vi "Begin.vi"(8 "error in":errorcluster) -> (0 "error out":errorcluster)   [LabVIEW 2018]
doc: "Called before other user functions, this VI is expected to open initial I/O refnums, load in file data, and do all program initialization. Notice that the <B>error out</B> terminal is simply used for data flow. Wiring it to other structures or subVIs ensures that this VI runs first."
uses:
  <vilib>/Rock Robotics/WPI/DriverStation/WPI_DriverStationRobotMode2.ctl
  <vilib>/Rock Robotics/WPI/Joystick/WPI_JoystickDeviceEnum.ctl
  Robot Global Data.vi
  <vilib>/Rock Robotics/Network Tables/NT Write String Array.vi
  <vilib>/Rock Robotics/WPI/RobotDrive/WPI_RobotDriveOpen2MotorWithExistingMotors.vi
  <vilib>/Rock Robotics/SystemInterfaces/DIO/FPGA_DIOPWMChannel.ctl
  <vilib>/Rock Robotics/WPI/SafetyOutput/WPI_SafetyOutputConfigMenu.ctl
  <vilib>/Rock Robotics/WPI/RobotDrive/WPI_RobotDriveOpen4MotorWithTalon.vi
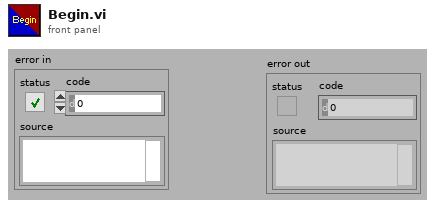
[diagram p1: front panel]
types:
  T1 = enum16{"Talon-RightDrive", "Victor-Right1", "Victor-Right2", "Talon-RHabArm", "Talon-RHabSlide", "Victor-CargoIntake1", "Victor-CargoIntake2", "Talon-CargoRotate", "Empty1", "Empty2", "Victor-HabWheel", "Talon-LHabSlide", "Talon-LHabArm", "Victor-Left1", "Victor-Left2", "Talon-LeftDrive"}
  T2 = typedef "WPI_JoystickDeviceEnum.ctl" = enum16{"USB 0", "USB 1", "USB 2", "USB 3", "USB 4", "USB 5"}
  T3 = typedef "WPI_DriverStationRobotMode2.ctl" = enum16{"Autonomous Disabled", "Autonomous Enabled", "Teleop Disabled", "Teleop Enabled", "Disconnected", "Finish", "Test Disabled", "Test Enabled", "Emergency Stopped"}
  T4 = typedef "CTRE_CANifier_PWMChannel.ctl" = enum16{"PWMChannel0", "PWMChannel1", "PWMChannel2", "PWMChannel3"}
  T5 = typedef "CTRE_CANifier_DeviceRef.ctl" = cluster{"DeviceStatus":errorcluster, "Device Number":u8, "Handle":u64, "UsageFrame":u32, "Library Path":path}
  T6 = typedef "FPGA_DIOPWMChannel.ctl" = enum8{"PWM 0", "PWM 1", "PWM 2", "PWM 3", "PWM 4", "PWM 5", "PWM 6", "PWM 7", "PWM 8", "PWM 9", "PWM MXP 0", "PWM MXP 1", "PWM MXP 2", "PWM MXP 3", "PWM MXP 4", "PWM MXP 5", "PWM MXP 6", "PWM MXP 7", "PWM MXP 8", "PWM MXP 9", "Invalid"}
  T7 = typedef "WPI_SafetyOutputConfigMenu.ctl" = enum16{"Enable", "Disable"}
  T8 = typedef "WPI_RobotDriveDevRef.ctl" = cluster{"DevStatus":errorcluster, "Motors[]":T9[], "Square Inputs":bool, "Max Output":dbl}
  T9 = typedef "WPI_MotorControlDeviceRef.ctl" = cluster{"DeviceStatus":errorcluster, "Type":T10, "PWM":cluster{"PWM Channel":T6, "DeadBand":T11}, "CAN":cluster{"Device Number":u8, "SetOutput VI Ref":variant, "GetOutput VI Ref":variant, "Enable VI Ref":variant, "Disable VI Ref":variant, "Data":variant}, "Invert":bool, "DIO PWM":cluster{"PWM \"Enable\" Channel":T6, "DIOChannel":T12, "PWM Rate":dbl}}
  T10 = typedef "WPI_MotorControlType.ctl" = enum16{"PWM", "CAN", "DIO PWM"}
  T11 = typedef "WPI_PWMDeadband.ctl" = cluster{"Name":string, "maxPositivePwm":i32, "minPositivePwm":i32, "centerPwm":i32, "maxNegativePwm":i32, "minNegativePwm":i32, "angularRange":u16}
  T12 = typedef "FPGA_DIOChannel.ctl" = enum8{"DIO 0", "DIO 1", "DIO 2", "DIO 3", "DIO 4", "DIO 5", "DIO 6", "DIO 7", "DIO 8", "DIO 9", "DIO MXP 0", "DIO MXP 1", "DIO MXP 2", "DIO MXP 3", "DIO MXP 4", "DIO MXP 5", "DIO MXP 6", "DIO MXP 7", "DIO MXP 8", "DIO MXP 9", "DIO MXP 10", "DIO MXP 11", "DIO MXP 12", "DIO MXP 13", "DIO MXP 14", "DIO MXP 15", "SPI Port CS1", "SPI Port CS2", "SPI Port CS3", "SPI Port MISO", "SPI Port MOSI", "Invalid"}
  T13 = typedef "WPI_JoystickDevRef.ctl" = cluster{"Device":T2}
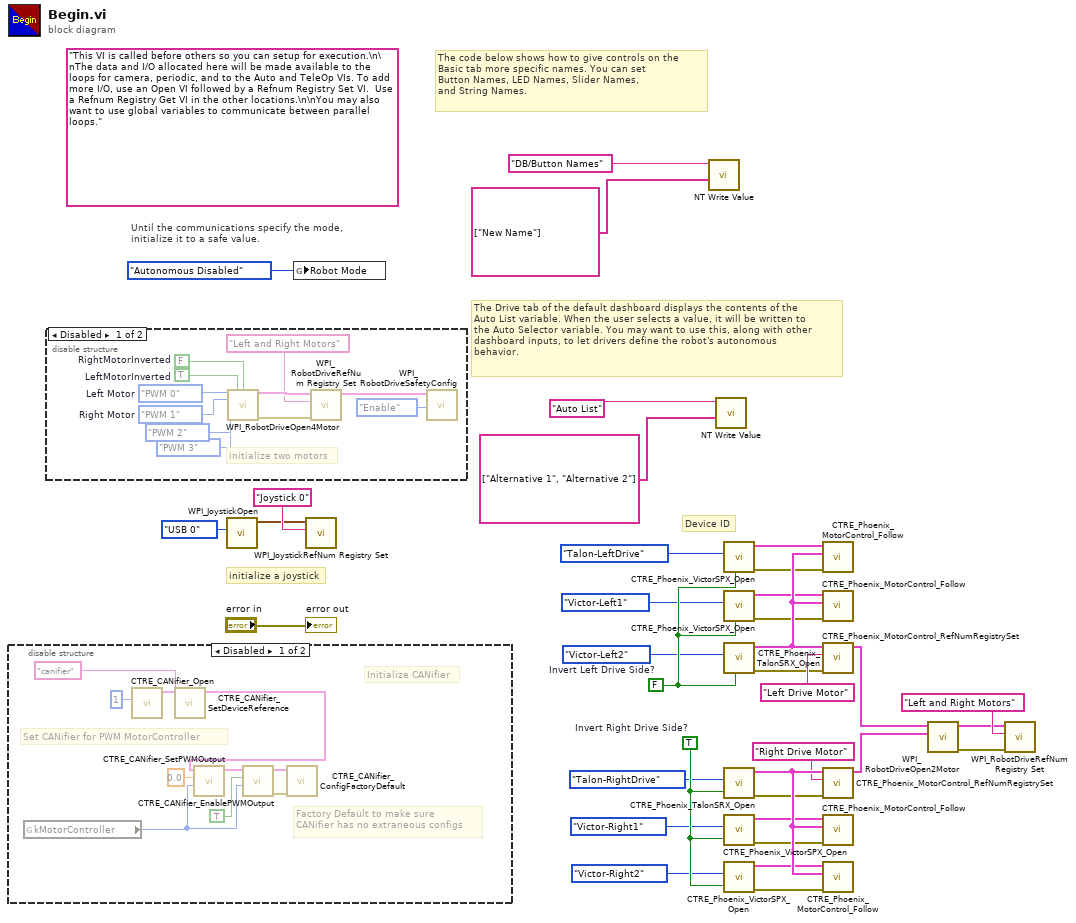
[diagram p0: block diagram]
diagram:
  w27 = FALSE  # Invert Left Drive Side?
  w26 = TRUE  # Invert Right Drive Side?
  (unwired) "This VI is called before others so you can setup for execution.\n\nThe data and I/O allocated here will be made available to the loops for camera, periodic, and to the Auto and TeleOp VIs. To add more I/O, use an Open VI followed by a Refnum Registry Set VI.  Use a Refnum Registry Get VI in the other locations.\n\nYou may also want to use global variables to communicate between parallel loops."
  # "Device ID"
  # "The Drive tab of the default dashboard displays the contents of the\nAuto List variable. When the user selects a value, it will be written to\nthe Auto Selector variable. You may want to use this, along with other\ndashboard inputs, to let drivers define the robot's autonomous\nbehavior."
  # "The code below shows how to give controls on the\nBasic tab more specific names. You can set\nButton Names, LED Names, Slider Names,\nand String Names."
  # "initialize a joystick"
  # "Until the communications specify the mode,\ninitialize it to a safe value."
  n1 = disable-structure shown="Disabled" {
    frame Disabled {
      # "Initialize CANifier"
      # "Factory Default to make sure\nCANifier has no extraneous configs"
      # "Set CANifier for PWM MotorController"
      n2 = global read "Robot Global Data.vi" "kMotorController"() -> (w42:T4)
      n3 = call <vilib>:"CTRE_CANifier_Open.vi"("Device Number"=u8 1) -> ("CANifierDevRef"=w39:T5)  [unwired: 9 in, 1 out]
      n4 = call <vilib>:"CTRE_CANifier_SetDeviceReference.vi"("refnum name"="canifier", "CANifierDevRef"=w39) -> ("CANifierDevRef"=w37:T5)  [unwired: 8 in, 1 out]
      n5 = call <vilib>:"CTRE_CANifier_SetPWMOutput.vi"("PWMChannel"=w42, "Duty Cycle"=0.0, "CANifierDevRef"=w37) -> ("CANifierDevRef"=w41:T5)  [unwired: 7 in, 1 out]
      n6 = call <vilib>:"CTRE_CANifier_EnablePWMOutput.vi"("PWMChannel"=w42, "Enable?"=TRUE, "CANifierDevRef"=w41) -> ("error out"=w45:errorcluster, "CANifierDevRef"=w46:T5)  [unwired: 7 in]
      n7 = call <vilib>:"CTRE_CANifier_ConfigFactoryDefault.vi"("error in"=w45, "CANifierDevRef"=w46) -> ()  [unwired: 8 in, 2 out]
    }
    frame Enabled {
    }
  }
  n8 = disable-structure shown="Disabled" {
    frame Disabled {
      w51 = FPGA_DIOPWMChannel."PWM 1"  # Right Motor
      w52 = FPGA_DIOPWMChannel."PWM 0"  # Left Motor
      w56 = TRUE  # LeftMotorInverted
      w57 = FALSE  # RightMotorInverted
      # "initialize two motors"
      n9 = call-poly <vilib>:"WPI_RobotDriveOpen4Motor.vi"("Rear Left Motor"=w52, "Rear Left Motor Inverted"=w56, "Rear Right Motor Inverted"=w57, "Rear Right Motor"=w51, "Front Left Motor"=FPGA_DIOPWMChannel."PWM 2", "Front Right Motor"=FPGA_DIOPWMChannel."PWM 3") -> ("RobotDriveDevRef"=w55:T8, "error out"=w53:errorcluster)  [unwired: 8 in]
      n10 = call <vilib>:"WPI_RobotDriveRefNum Registry Set.vi"("error in (no error)"=w53, "refnum name"="Left and Right Motors", "RobotDriveDevRef"=w55) -> ("RobotDriveDevRef"=w50:T8)  [unwired: 1 in, 7 out]
      n11 = call <vilib>:"WPI_RobotDriveSafetyConfig.vi"("mode"=WPI_SafetyOutputConfigMenu."Enable", "RobotDriveDevRef"=w50) -> ()  [unwired: 8 in, 2 out]
    }
    frame Enabled {
    }
  }
  n12 = call <vilib>:"WPI_JoystickOpen.vi"("JoystickDevice"=WPI_JoystickDeviceEnum."USB 0") -> ("JoystickDevRef"=w34:T13)  [unwired: 10 in]
  n13 = global write "Robot Global Data.vi" "Robot Mode"(WPI_DriverStationRobotMode2."Autonomous Disabled" ("Robot Mode")) -> ()
  n14 = call <vilib>:"WPI_JoystickRefNum Registry Set.vi"("refnum name"="Joystick 0", "JoystickDevRef"=w34) -> ()  [unwired: 8 in, 2 out]
  n15 = call-poly <vilib>:"NT Write Value.vi"("String Array"=string[] ["New Name"], "Name"="DB/Button Names") -> ()  [unwired: 9 in, 1 out]
  n16 = call-poly <vilib>:"NT Write Value.vi"("String Array"=string[] ["Alternative 1", "Alternative 2"], "Name"="Auto List") -> ()  [unwired: 9 in, 1 out]
  n17 = call <vilib>:"CTRE_Phoenix_VictorSPX_Open.vi"("Invert"=w27, "Device Number"=T1."Talon-LeftDrive" ("PWMChannel")) -> ("error out"=w17:errorcluster, "CAN Talon SRX Ref"=w18:T9)  [unwired: 8 in]
  n18 = call <vilib>:"CTRE_Phoenix_VictorSPX_Open.vi"("Invert"=w27, "Device Number"=T1."Victor-Left1" ("PWMChannel")) -> ("error out"=w16:errorcluster, "CAN Talon SRX Ref"=w19:T9)  [unwired: 8 in]
  n19 = call <vilib>:"CTRE_Phoenix_TalonSRX_Open.vi"("Invert"=w27, "Device Number"=T1."Victor-Left2" ("PWMChannel")) -> ("error out"=w7:errorcluster, "CAN Talon SRX Ref"=w20:T9)  [unwired: 8 in]
  n20 = call <vilib>:"CTRE_Phoenix_TalonSRX_Open.vi"("Invert"=w26, "Device Number"=T1."Talon-RightDrive" ("PWMChannel")) -> ("error out"=w8:errorcluster, "CAN Talon SRX Ref"=w15:T9)  [unwired: 8 in]
  n21 = call <vilib>:"CTRE_Phoenix_VictorSPX_Open.vi"("Invert"=w26, "Device Number"=T1."Victor-Right1" ("PWMChannel")) -> ("error out"=w11:errorcluster, "CAN Talon SRX Ref"=w12:T9)  [unwired: 8 in]
  n22 = call <vilib>:"CTRE_Phoenix_VictorSPX_Open.vi"("Invert"=w26, "Device Number"=T1."Victor-Right2" ("PWMChannel")) -> ("error out"=w14:errorcluster, "CAN Talon SRX Ref"=w13:T9)  [unwired: 8 in]
  n23 = call <vilib>:"CTRE_Phoenix_MotorControl_Follow.vi"("error in (no error)"=w17, "Master Controller to Follow"=w20, "PhoenixMotorControlDevRef"=w18) -> ()  [unwired: 7 in, 2 out]
  n24 = call <vilib>:"CTRE_Phoenix_MotorControl_Follow.vi"("error in (no error)"=w16, "Master Controller to Follow"=w20, "PhoenixMotorControlDevRef"=w19) -> ()  [unwired: 7 in, 2 out]
  n25 = call <vilib>:"CTRE_Phoenix_MotorControl_RefNumRegistrySet.vi"("error in (no error)"=w7, "refnum name"="Left Drive Motor", "PhoenixMotorControlDevRef"=w20) -> ("PhoenixMotorControlDevRef"=w21:T9)  [unwired: 7 in, 1 out]
  n26 = call <vilib>:"CTRE_Phoenix_MotorControl_RefNumRegistrySet.vi"("error in (no error)"=w8, "refnum name"="Right Drive Motor", "PhoenixMotorControlDevRef"=w15) -> ("PhoenixMotorControlDevRef"=w22:T9)  [unwired: 7 in, 1 out]
  n27 = call <vilib>:"CTRE_Phoenix_MotorControl_Follow.vi"("error in (no error)"=w11, "Master Controller to Follow"=w15, "PhoenixMotorControlDevRef"=w12) -> ()  [unwired: 7 in, 2 out]
  n28 = call <vilib>:"CTRE_Phoenix_MotorControl_Follow.vi"("error in (no error)"=w14, "Master Controller to Follow"=w15, "PhoenixMotorControlDevRef"=w13) -> ()  [unwired: 7 in, 2 out]
  n29 = call-poly <vilib>:"WPI_RobotDriveOpen2Motor.vi"("Right Motor Dev Ref"=w22, "Left Motor Dev Ref"=w21) -> ("error out"=w23:errorcluster, "RobotDriveDevRef"=w24:T8)  [unwired: 8 in]
  n30 = call <vilib>:"WPI_RobotDriveRefNum Registry Set.vi"("error in (no error)"=w23, "refnum name"="Left and Right Motors", "RobotDriveDevRef"=w24) -> ()  [unwired: 7 in, 2 out]
  "error out" <- "error in"
